vi "test_UDP_UDP Clear Error.vi"(8 "error in (no error)":errorcluster, 11 "TestCase in":refnum<class "Ethernet Protocol Tests.lvclass">) -> (0 "error out":errorcluster, 3 "TestCase out":refnum<class "Ethernet Protocol Tests.lvclass">)   [LabVIEW 2019, in "Ethernet Protocol Tests.lvclass"]
uses:
  Ethernet Protocol Tests.lvclass
  UDP/UDP.lvclass
  UDP/UDP.lvclass/UDP.ctl
  UDP/Data Access/Write Local IP Address.vi
  UDP/Data Access/Write Target IP Address.vi
  UDP/Data Access/Write Local Port.vi
  UDP/Data Access/Write Target Port.vi
  <vilib>/Utility/error.llb/Error Cluster From Error Code.vi
  <vilib>/ErrorRing/Error Ring.xnode
  <vilib>/addons/_JKI Toolkits/VI Tester/TestCase.llb/TestCase.lvclass
  C:/Program Files (x86)/National Instruments/LabVIEW 2019/vi.lib/addons/_JKI Toolkits/VI Tester/TestCase.llb/TestCase.lvclass
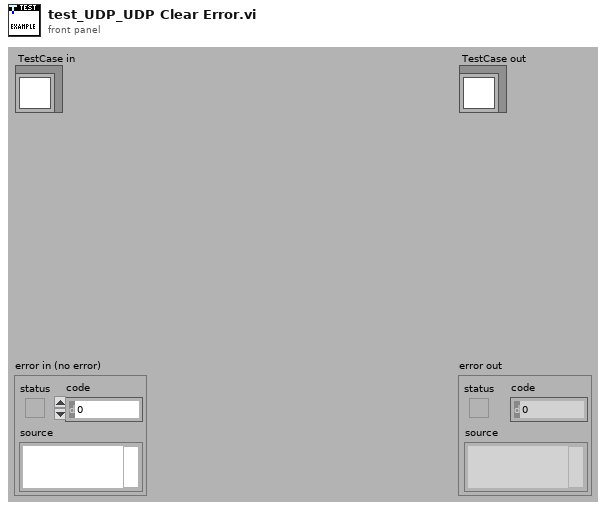
[diagram p1: front panel]
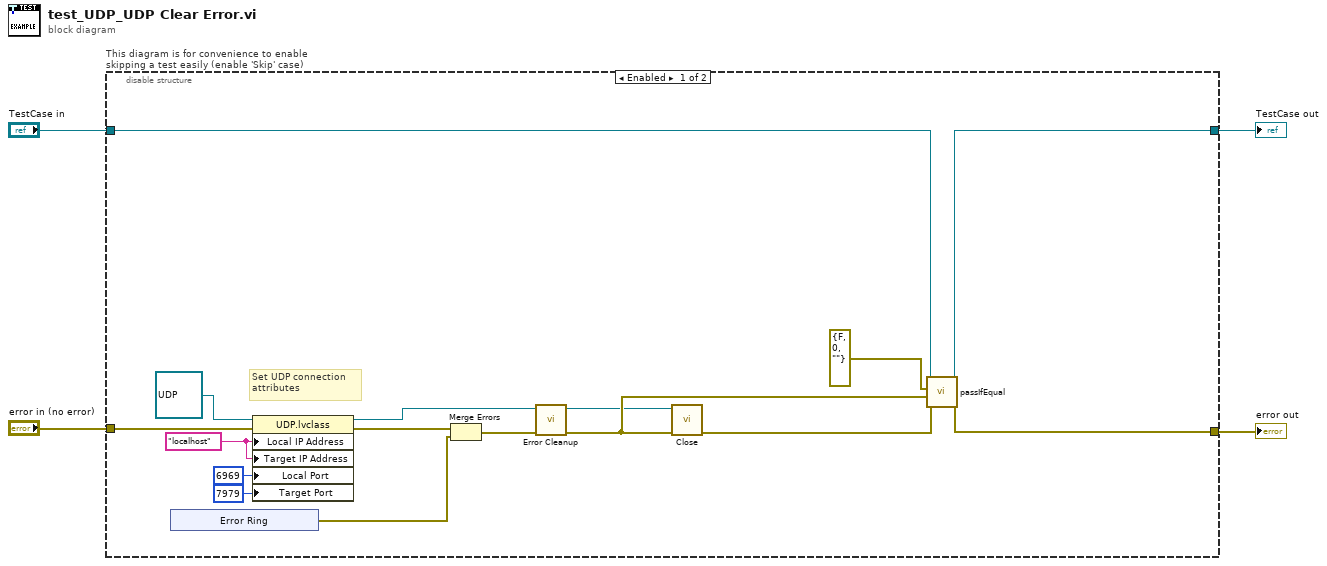
[diagram p0: block diagram]
diagram:
  n1 = disable-structure "This diagram is for convenience to enable skipping a test easily (enable 'Skip' case)" shown="Enabled" {
    disable-tunnel: "TestCase in" -> [w20 w29]
    disable-tunnel: [w19 w27] -> w1
    disable-tunnel: [w18 w28] -> w3
    disable-tunnel: "error in (no error)" -> [w16 w26]
    frame Enabled {
      w15 = "localhost" ("Local IP Address")
      # "Set UDP connection \nattributes"
      n2 = xnode "Error Ring"() -> ("error out"=w10:errorcluster)
      n3 = property class="UDP.lvclass"(reference=refnum<class "UDP.lvclass"> refnum ("Protocols.lvlib:UDP.lvclass"), error in=w16, "Local IP Address"=w15, "Target IP Address"=w15, "Local Port"=u16 6969, "Target Port"=u16 7979) -> (reference out=w9:refnum<class "UDP.lvclass">, error out=w12:errorcluster)
      n4 = Merge Errors(w12, w10) -> (w11:errorcluster)
      n5 = call-dynamic "Error Cleanup.vi"("error in (no error)"=w11, "UDP in"=w9) -> ("error out"=w6:errorcluster, "UDP out"=w5:refnum<class "UDP.lvclass">)  [unwired: 8 in]
      n6 = call-dynamic "Close.vi"("error in (no error)"=w6, "UDP in"=w5) -> ("error out"=w7:errorcluster)  [unwired: 8 in, 1 out]
      n7 = call-dynamic "passIfEqual.vi"("error in (no error)"=w7, "y"=w6, "x"=errorcluster {"status"=FALSE, "code"=0, "source"=""} ("error constant"), "TestCase in"=w20) -> ("error out"=w18:errorcluster, "TestCase out"=w19:refnum<class "Ethernet Protocol Tests.lvclass">)  [unwired: 6 in]
    }
    frame Disabled {
      # "skip test result while test is under development"
      n8 = call <vilib>:"skip.vi"("error in (no error)"=w26, "TestCase in"=w29) -> ("error out"=w28:errorcluster, "TestCase out"=w27:refnum<class "Ethernet Protocol Tests.lvclass">)  [unwired: 8 in]
    }
  }
  "error out" <- w3
  "TestCase out" <- w1
